vi "校准信息转u16数组.vi"(11 "关键参数":T1(array[cluster])) -> (3 "添加的数组":u16[](array[numeric]))   [LabVIEW 2016, in "MB SLAVE.lvlib"]
uses:
  MB SLAVE.lvlib
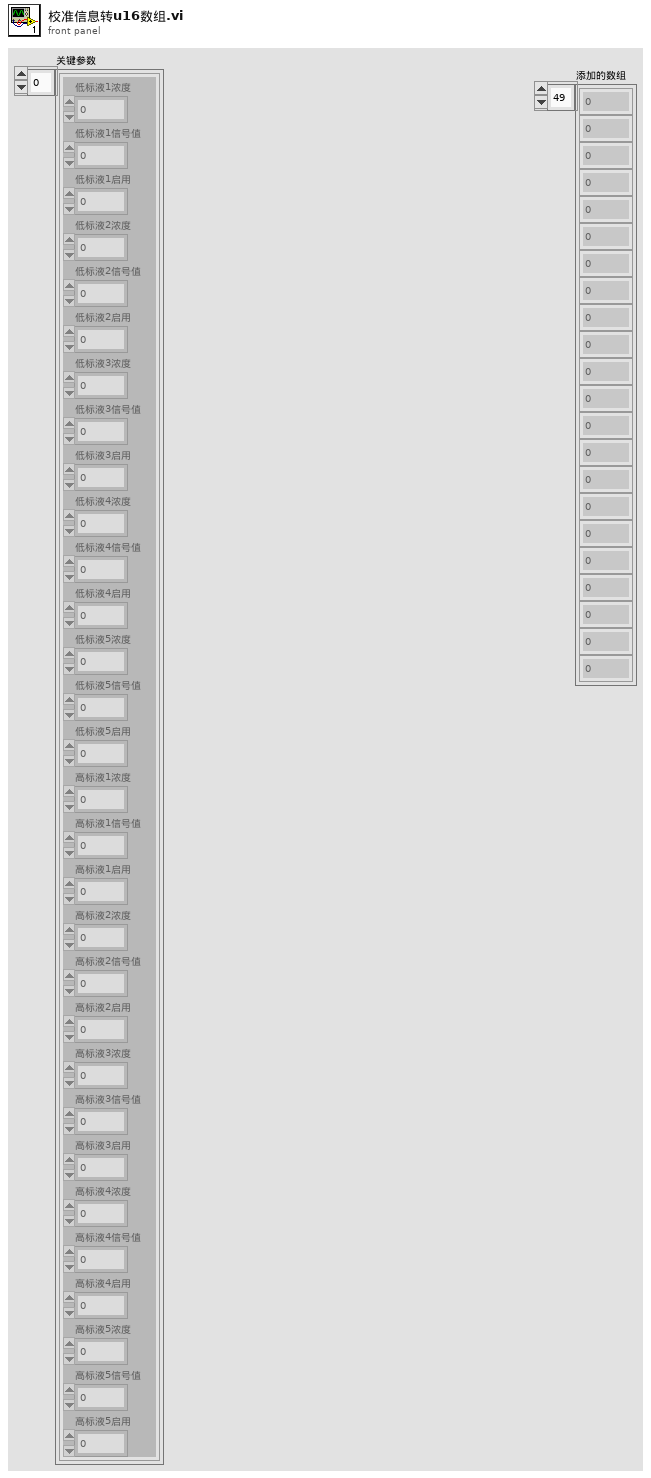
[diagram p1: front panel]
types:
  T1 = cluster{"低标液1浓度":dbl, "低标液1信号值":dbl, "低标液1启用":u16, "低标液2浓度":dbl, "低标液2信号值":dbl, "低标液2启用":u16, "低标液3浓度":dbl, "低标液3信号值":dbl, "低标液3启用":u16, "低标液4浓度":dbl, "低标液4信号值":dbl, "低标液4启用":u16, "低标液5浓度":dbl, "低标液5信号值":dbl, "低标液5启用":u16, "高标液1浓度":dbl, "高标液1信号值":dbl, "高标液1启用":u16, "高标液2浓度":dbl, "高标液2信号值":dbl, "高标液2启用":u16, "高标液3浓度":dbl, "高标液3信号值":dbl, "高标液3启用":u16, "高标液4浓度":dbl, "高标液4信号值":dbl, "高标液4启用":u16, "高标液5浓度":dbl, "高标液5信号值":dbl, "高标液5启用":u16}[]
  T2 = cluster{"低标液1浓度":dbl, "低标液1信号值":dbl, "低标液1启用":u16, "低标液2浓度":dbl, "低标液2信号值":dbl, "低标液2启用":u16, "低标液3浓度":dbl, "低标液3信号值":dbl, "低标液3启用":u16, "低标液4浓度":dbl, "低标液4信号值":dbl, "低标液4启用":u16, "低标液5浓度":dbl, "低标液5信号值":dbl, "低标液5启用":u16, "高标液1浓度":dbl, "高标液1信号值":dbl, "高标液1启用":u16, "高标液2浓度":dbl, "高标液2信号值":dbl, "高标液2启用":u16, "高标液3浓度":dbl, "高标液3信号值":dbl, "高标液3启用":u16, "高标液4浓度":dbl, "高标液4信号值":dbl, "高标液4启用":u16, "高标液5浓度":dbl, "高标液5信号值":dbl, "高标液5启用":u16}
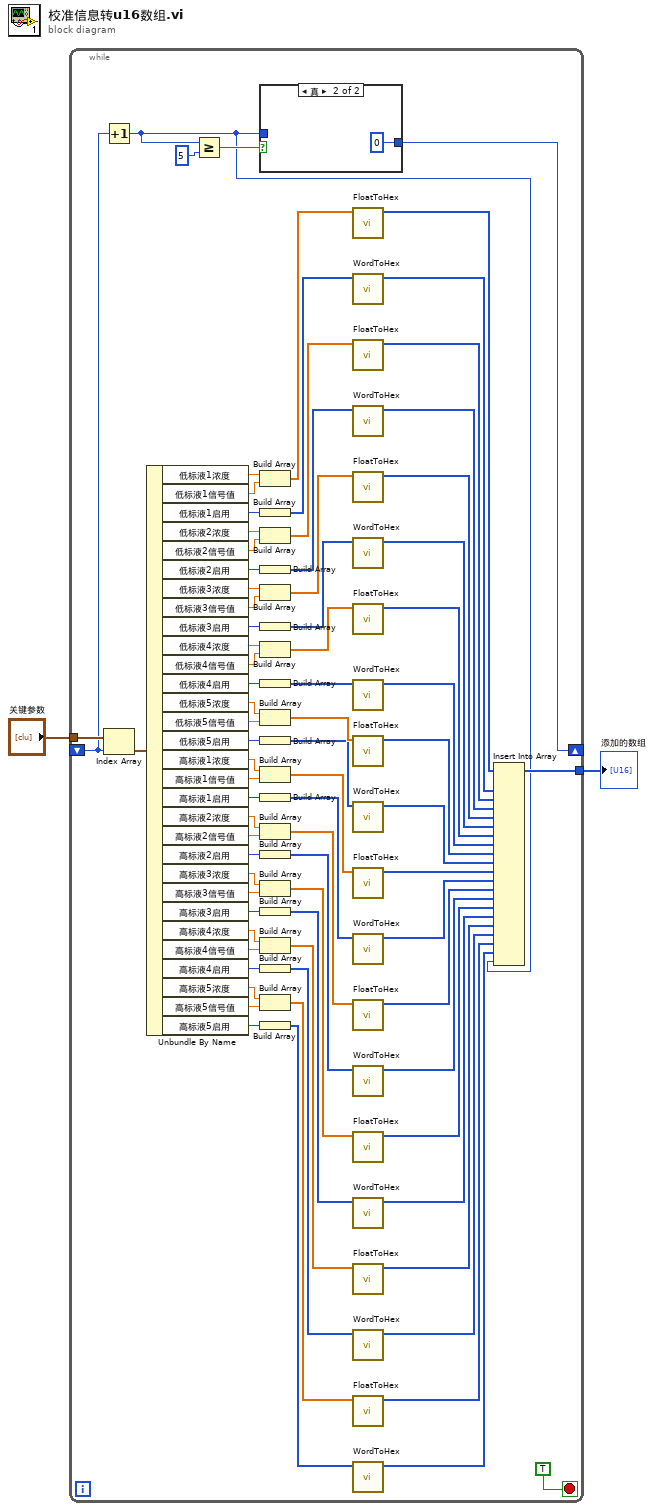
[diagram p0: block diagram]
diagram:
  n1 = while {
    tunnel: "关键参数" -> [w80]
    shift-right: [w73] -> _
    shift-left: _ -> [w77]
    tunnel: [w76] -> w1
    stop <- TRUE stop-if-true
    n2 = Increment(x=w77) -> (x+1=w3:u16)
    n3 = Index Array(array=w80, index=w77) -> (element=w79:T2)
    n4 = Unbundle By Name(w79) -> ("低标液1浓度"=w72:dbl, "低标液1信号值"=w71:dbl, "低标液1启用"=w68:u16, "低标液2浓度"=w65:dbl, "低标液2信号值"=w64:dbl, "低标液2启用"=w81:u16, "低标液3浓度"=w58:dbl, "低标液3信号值"=w57:dbl, "低标液3启用"=w56:u16, "低标液4浓度"=w50:dbl, "低标液4信号值"=w49:dbl, "低标液4启用"=w48:u16, "低标液5浓度"=w43:dbl, "低标液5信号值"=w42:dbl, "低标液5启用"=w41:u16, "高标液1浓度"=w36:dbl, "高标液1信号值"=w35:dbl, "高标液1启用"=w33:u16, "高标液2浓度"=w29:dbl, "高标液2信号值"=w28:dbl, "高标液2启用"=w27:u16, "高标液3浓度"=w20:dbl, "高标液3信号值"=w19:dbl, "高标液3启用"=w18:u16, "高标液4浓度"=w13:dbl, "高标液4信号值"=w12:dbl, "高标液4启用"=w11:u16, "高标液5浓度"=w10:dbl, "高标液5信号值"=w9:dbl, "高标液5启用"=w8:u16)
    n5 = Greater Or Equal?(x=w3, y=u16 5) -> (x >= y?=w74:bool)
    n6 = case shown="真" w74 {
      tunnel: [w82 u16 0] -> w73
      tunnel: w3 -> [w82 _]
      frame False {
      }
      frame True {
      }
    }
    n7 = Build Array(w72, w71) -> (w70:dbl[])
    n8 = Build Array(w68) -> (w67:u16[])
    n9 = Build Array(w65, w64) -> (w63:dbl[])
    n10 = Build Array(w81) -> (w62:u16[])
    n11 = Build Array(w58, w57) -> (w59:dbl[])
    n12 = Build Array(w56) -> (w55:u16[])
    n13 = Build Array(w50, w49) -> (w52:dbl[])
    n14 = Build Array(w48) -> (w51:u16[])
    n15 = Build Array(w43, w42) -> (w45:dbl[])
    n16 = Build Array(w41) -> (w44:u16[])
    n17 = Build Array(w36, w35) -> (w38:dbl[])
    n18 = Build Array(w33) -> (w37:u16[])
    n19 = Build Array(w29, w28) -> (w31:dbl[])
    n20 = Build Array(w27) -> (w30:u16[])
    n21 = Build Array(w20, w19) -> (w24:dbl[])
    n22 = Build Array(w18) -> (w23:u16[])
    n23 = Build Array(w13, w12) -> (w22:dbl[])
    n24 = Build Array(w11) -> (w21:u16[])
    n25 = Build Array(w10, w9) -> (w15:dbl[])
    n26 = Build Array(w8) -> (w14:u16[])
    n27 = call "FloatToHex.vi"("FLOAT"=w70) -> ("交织的数组"=w69:u16[])  [unwired: 10 in]
    n28 = call "WordToHex.vi"("WORD"=w67) -> ("数组"=w66:u16[])  [unwired: 10 in]
    n29 = call "FloatToHex.vi"("FLOAT"=w63) -> ("交织的数组"=w61:u16[])  [unwired: 10 in]
    n30 = call "WordToHex.vi"("WORD"=w62) -> ("数组"=w60:u16[])  [unwired: 10 in]
    n31 = call "FloatToHex.vi"("FLOAT"=w59) -> ("交织的数组"=w54:u16[])  [unwired: 10 in]
    n32 = call "WordToHex.vi"("WORD"=w55) -> ("数组"=w53:u16[])  [unwired: 10 in]
    n33 = call "FloatToHex.vi"("FLOAT"=w52) -> ("交织的数组"=w47:u16[])  [unwired: 10 in]
    n34 = call "WordToHex.vi"("WORD"=w51) -> ("数组"=w46:u16[])  [unwired: 10 in]
    n35 = call "FloatToHex.vi"("FLOAT"=w45) -> ("交织的数组"=w40:u16[])  [unwired: 10 in]
    n36 = call "WordToHex.vi"("WORD"=w44) -> ("数组"=w39:u16[])  [unwired: 10 in]
    n37 = call "FloatToHex.vi"("FLOAT"=w38) -> ("交织的数组"=w34:u16[])  [unwired: 10 in]
    n38 = call "WordToHex.vi"("WORD"=w37) -> ("数组"=w32:u16[])  [unwired: 10 in]
    n39 = call "FloatToHex.vi"("FLOAT"=w31) -> ("交织的数组"=w26:u16[])  [unwired: 10 in]
    n40 = call "WordToHex.vi"("WORD"=w30) -> ("数组"=w25:u16[])  [unwired: 10 in]
    n41 = call "FloatToHex.vi"("FLOAT"=w24) -> ("交织的数组"=w17:u16[])  [unwired: 10 in]
    n42 = call "WordToHex.vi"("WORD"=w23) -> ("数组"=w16:u16[])  [unwired: 10 in]
    n43 = call "FloatToHex.vi"("FLOAT"=w22) -> ("交织的数组"=w7:u16[])  [unwired: 10 in]
    n44 = call "WordToHex.vi"("WORD"=w21) -> ("数组"=w6:u16[])  [unwired: 10 in]
    n45 = call "FloatToHex.vi"("FLOAT"=w15) -> ("交织的数组"=w5:u16[])  [unwired: 10 in]
    n46 = call "WordToHex.vi"("WORD"=w14) -> ("数组"=w4:u16[])  [unwired: 10 in]
    n47 = Insert Into Array(array=w69, new element #1=w66, new element #2=w61, new element #3=w60, new element #4=w54, new element #5=w53, new element #6=w47, new element #7=w46, new element #8=w40, new element #9=w39, new element #10=w34, new element #11=w32, new element #12=w26, new element #13=w25, new element #14=w17, new element #15=w16, new element #16=w7, new element #17=w6, new element #18=w5, new element #19=w4, new element #20=w3) -> (w76:u16[])  [unwired: 1 in]
  }
  "添加的数组" <- w1
